vi "SVFA Compensate Phase for Time Delay.vi"   [LabVIEW 2017]
doc: "Compensates FFT and frequency response phase spectra for time delay. You can introduce time delays with the DUT, data acquisition hardware, and measurement analysis. Compensation in this VI is restricted to linear phase resulting from a pure time delay. Wire data to the <B>phase spectrum</B> input to determine the polymorphic instance to use or manually select the instance."
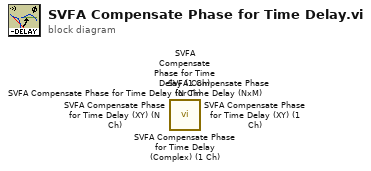
[diagram p0: block diagram]
diagram:
  n1 = call <vilib>:"SVFA Compensate Phase for Time Delay (Complex) (1 Ch).vi"() -> ()  [unwired: 18 in, 2 out]
  n2 = call <vilib>:"SVFA Compensate Phase for Time Delay (NxM).vi"() -> ()  [unwired: 16 in, 4 out]
  n3 = call <vilib>:"SVFA Compensate Phase for Time Delay (XY) (N Ch).vi"() -> ()  [unwired: 16 in, 4 out]
  n4 = call <vilib>:"SVFA Compensate Phase for Time Delay (XY) (1 Ch).vi"() -> ()  [unwired: 16 in, 4 out]
  n5 = call <vilib>:"SVFA Compensate Phase for Time Delay (N Ch).vi"() -> ()  [unwired: 16 in, 4 out]
  n6 = call <vilib>:"SVFA Compensate Phase for Time Delay (1 Ch).vi"() -> ()  [unwired: 16 in, 4 out]
